vi "Send Msg and Wait on Response.vi"(6 "Priority Message? (F)":bool, 7 "timeout in ms (5000)":i32=5000, 8 "error in (no error)":errorcluster, 9 "Message Data":variant, 10 "Message":string, 11 "Subscription References":T1) -> (0 "error out":errorcluster)   [LabVIEW 2018]
uses:
  controls/Subscriber Comms Refs.ctl
  Message Queue/Message Cluster.ctl
  Message Queue/Enqueue Message (Single).vi
  Message Queue/Message Queue.lvlib
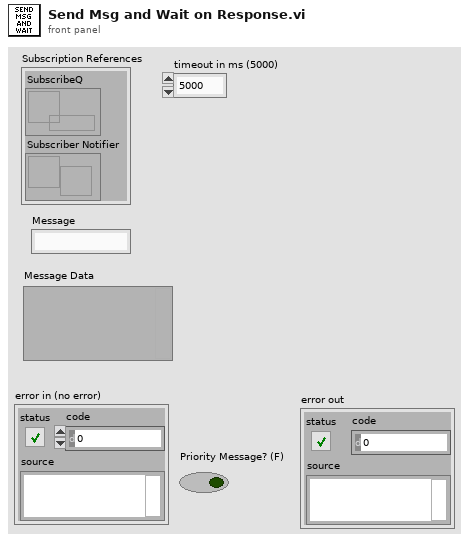
[diagram p1: front panel]
types:
  T1 = typedef "Subscriber Comms Refs.ctl" = cluster{"SubscribeQ":refnum<queue>, "Subscriber Notifier":refnum<notifier>}
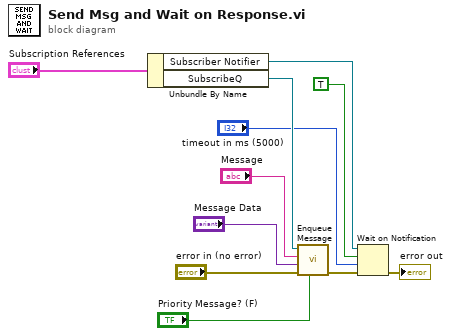
[diagram p0: block diagram]
diagram:
  n1 = Unbundle By Name("Subscription References") -> ("Subscriber Notifier"=w3:refnum<notifier>, "SubscribeQ"=w11:refnum<queue>)
  n2 = call-poly "Enqueue Message.vi"("Priority Message? (F)"="Priority Message? (F)", "error in (no error)"="error in (no error)", "Message Data"="Message Data", "Message"="Message", "Message Queue"=w11) -> ("error out"=w7:errorcluster)  [unwired: 5 in, 1 out]
  n3 = Wait on Notification(notifier=w3, ignore previous (F)=TRUE, timeout in ms (-1)="timeout in ms (5000)", error in (no error)=w7) -> (error out=→"error out":errorcluster)  [unwired: 3 out]
